vi "Post-Build Action.vi"(5 "Files Generated by Build":path[](array[path]), 6 "Top Level/Always Included VIs":path[](array[path]), 7 "Destination Path":path, 8 "error in (no error)":errorcluster, 9 "Target Name":string, 10 "Build Specification Name":string, 11 "Project Path":path) -> (0 "error out":errorcluster)   [LabVIEW 2017, in "Debug Server.lvclass"]
uses:
  Debug Server.lvclass
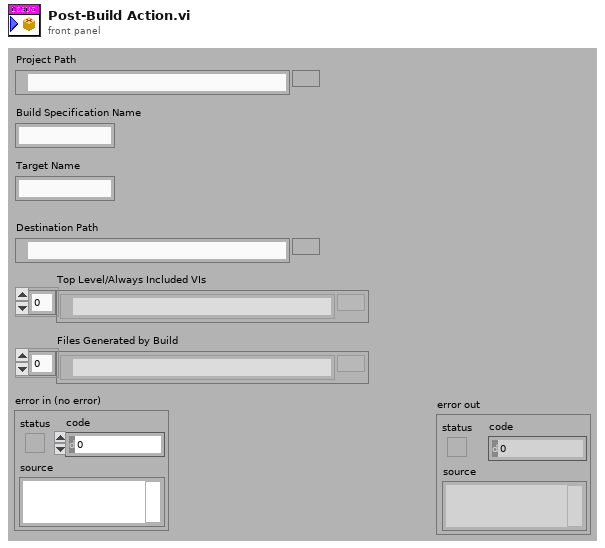
[diagram p1: front panel]
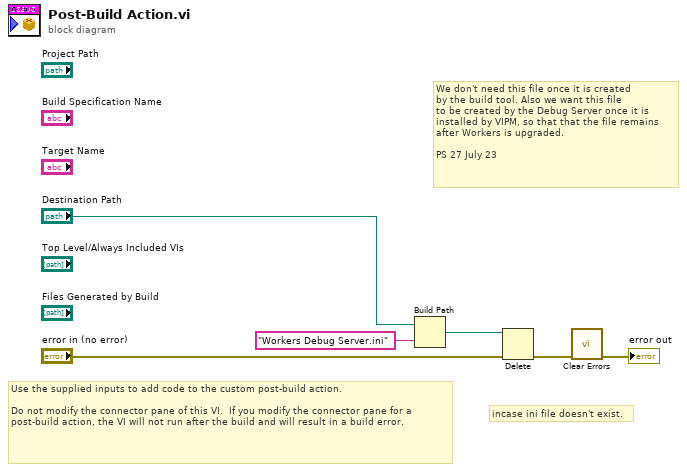
[diagram p0: block diagram]
diagram:
  # "incase ini file doesn't exist."
  # "We don't need this file once it is created \nby the build tool. Also we want this file\nto be created by the Debug Server once it is\ninstalled by VIPM, so that that the file remains\nafter Workers is upgraded.\n\nPS 27 July 23"
  # "Use the supplied inputs to add code to the custom post-build action.\n\nDo not modify the connector pane of this VI.  If you modify the connector pane for a post-build action, the VI will not run after the build and will result in a build error."
  n1 = Build Path(base path="Destination Path", name or relative path="Workers Debug Server.ini") -> (appended path=w5:path)
  n2 = Delete(path (use dialog)=w5, error in="error in (no error)") -> (error out=w4:errorcluster)  [unwired: 3 in, 2 out]
  n3 = call <vilib>:"Clear Errors.vi"("error in (no error)"=w4) -> ("error out"=→"error out":errorcluster)  [unwired: 5 in, 1 out]
